vi "write_params.vi"(8 "error in (no error)":errorcluster, 10 "params":T1={"n_components"=1.0, "covariance_type"="full", "tol"=0.001, "reg_covar"=1e-06, "max_iter"=100.0, "n_init"=1.0, "init_params"="kmeans", "weights_init"={"weights_init_type"="None", "weights_init_list"=[]}, "means_init"={"means_init_type"="None", "means_init_list"=[]}, "precisions_init"={"precisions_init_type"="None", "precisions_init_list"=[]}, "random_state"=0.0, "warm_start"=FALSE, "verbose"=0.0, "verbose_interval"=10.0}, 11 "GaussianMixture in":refnum<class "GaussianMixture.lvclass">) -> (0 "error out":errorcluster, 3 "GaussianMixture out":refnum<class "GaussianMixture.lvclass">)   [LabVIEW 2020, in "GaussianMixture.lvclass"]
uses:
  GaussianMixture.lvclass
  Controls/gaussian_mixture_params.ctl
  GaussianMixture.lvclass/GaussianMixture.ctl
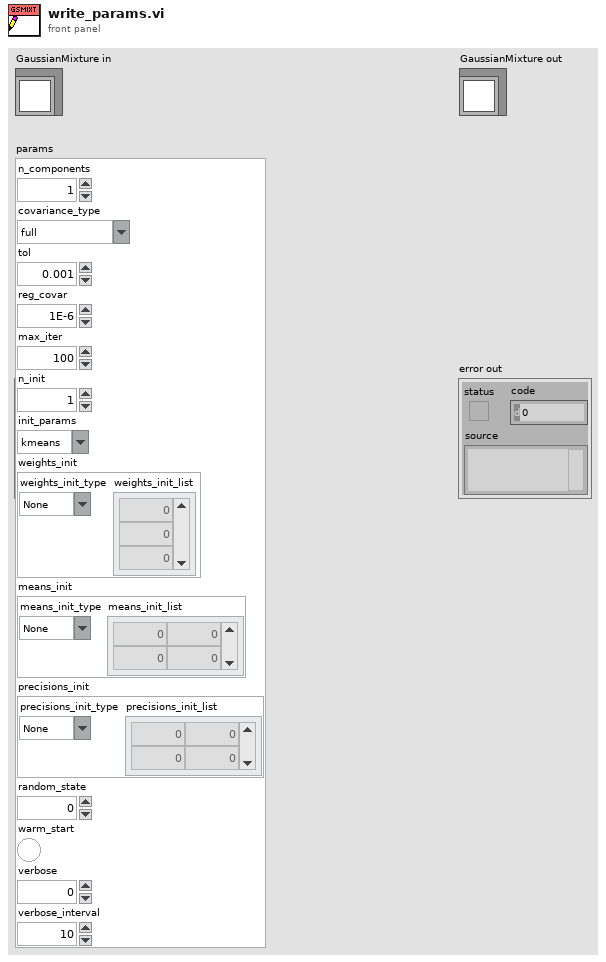
[diagram p1: front panel]
types:
  T1 = typedef "gaussian_mixture_params.ctl" = cluster{"n_components":dbl, "covariance_type":string, "tol":dbl, "reg_covar":dbl, "max_iter":dbl, "n_init":dbl, "init_params":string, "weights_init":cluster{"weights_init_type":string, "weights_init_list":dbl[]}, "means_init":cluster{"means_init_type":string, "means_init_list":dbl[][]}, "precisions_init":cluster{"precisions_init_type":string, "precisions_init_list":dbl[][]}, "random_state":dbl, "warm_start":bool, "verbose":dbl, "verbose_interval":dbl}
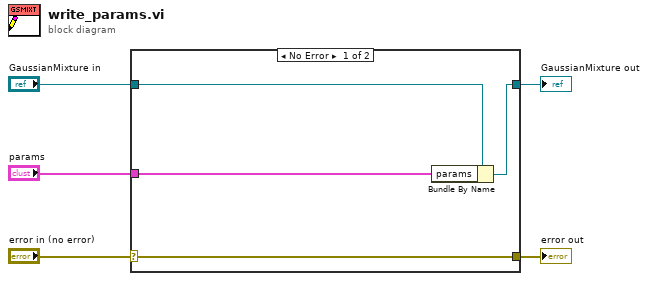
[diagram p0: block diagram]
diagram:
  n1 = case shown="No Error" "error in (no error)" {
    selector: "error in (no error)" -> [w9 w10]
    tunnel: [w9 w10] -> w4
    tunnel: [w7 w11] -> w2
    tunnel: "GaussianMixture in" -> [w8 w11]
    tunnel: "params" -> [w6 _]
    frame No Error {
      n2 = Bundle By Name(cluster=w8, "params"=w6) -> (w7:refnum<class "GaussianMixture.lvclass">)
    }
    frame Error {
    }
  }
  "error out" <- w4
  "GaussianMixture out" <- w2
